vi "Handle Last Ack Core.vi"(4 "error in (no error)":errorcluster, 6 "Last Ack":refnum<class "Last Ack.lvclass">, 7 "WebSocket Service Actor in":refnum<class "WebSocket Service.lvclass">) -> (0 "error out":errorcluster, 3 "WebSocket Service Actor out":refnum<class "WebSocket Service.lvclass">)   [LabVIEW 2021, in "WebSocket Actors.lvlib" / "WebSocket Service.lvclass"]
doc: "(<B>Filename</B>: Actor Framework.lvlib:Actor.lvclass:Handle Last Ack Core.vi)\n\nDefines how the caller actor responds to the Last Ack message from a nested actor. The Last Ack message is the final message a nested actor sends to its caller before it shuts down. The message contains information about the final state of the nested actor.\n\nBy default, this method does nothing except return any error the nested actor sent. A descendant class may override this method to define behavior."
uses:
  WebSocket Service.lvclass
  <vilib>/ActorFramework/LastAck/Last Ack.lvclass
  WebSocket Connection/WebSocket Connection.lvclass
  <vilib>/ActorFramework/LastAck/Last Ack.lvclass/Last Ack.ctl
  WebSocket Service.lvclass/WebSocket Service.ctl
  WebSocket Connection/WebSocket Connection.lvclass/WebSocket Connection.ctl
  <vilib>/ActorFramework/Report Error Msg/Report Error Msg.lvclass/Report Error Msg.ctl
  <vilib>/ActorFramework/Message Enqueuer/Message Enqueuer.lvclass/Message Enqueuer.ctl
  WebSocket Connection/properties/Read Peer ID.vi
  <vilib>/ActorFramework/Message Enqueuer/Enqueue.vi
  <vilib>/ActorFramework/Report Error Msg/Report Error Msg.lvclass
  C:/Program Files/National Instruments/LabVIEW 2021/vi.lib/ActorFramework/Message/Message.lvclass
  <vilib>/Utility/LVClass/Get LV Class Name.vi
  <resource>/AFDebug/Generate Trace for Message.vi
  <vilib>/ActorFramework/Message Priority Queue/Priority Enqueue.vi
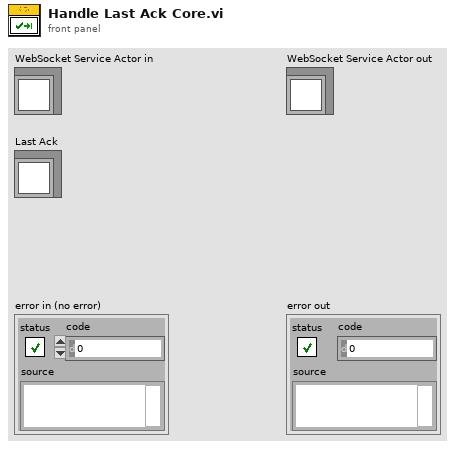
[diagram p1: front panel]
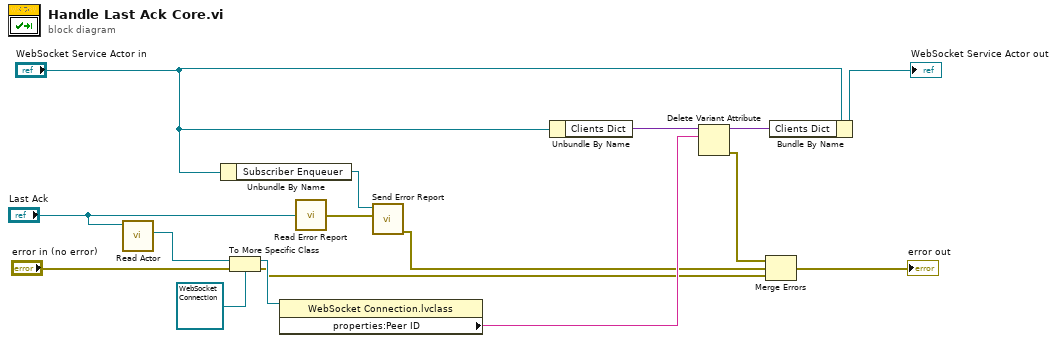
[diagram p0: block diagram]
diagram:
  n1 = call <vilib>:"Read Actor.vi"("Last Ack"="Last Ack") -> ("Actor"=w16:refnum<class "Actor.lvclass">)  [unwired: 10 in]
  n2 = Unbundle By Name("WebSocket Service Actor in") -> ("Subscriber Enqueuer"=w4:refnum<class "Message Enqueuer.lvclass">)
  n3 = To More Specific Class(target class=refnum<class "WebSocket Connection.lvclass"> refnum ("WebSocket Actors.lvlib:WebSocket Connection.lvclass"), reference=w16, error in="error in (no error)") -> (specific class reference=w15:refnum<class "WebSocket Connection.lvclass">, error out=w8:errorcluster)
  n4 = property class="WebSocket Connection.lvclass"(reference=w15) -> ("properties:Peer ID"=w9:string)  [unwired: 1 in, 2 out]
  n5 = call <vilib>:"Read Error Report.vi"("Last Ack"="Last Ack") -> ("error report"=w5:errorcluster)
  n6 = call <vilib>:"Send Error Report.vi"("Error From Sender"=w5, "Message Enqueuer"=w4) -> ("error out"=w3:errorcluster)  [unwired: 9 in]
  n7 = Unbundle By Name("WebSocket Service Actor in") -> ("Clients Dict"=w11:variant)
  n8 = Delete Variant Attribute(6:w9, 7:w11) -> (0:w2:errorcluster, 3:w10:variant)  [unwired: 1 in, 1 out]
  n9 = Merge Errors(w2, w3, w8) -> (→"error out":errorcluster)
  n10 = Bundle By Name(cluster="WebSocket Service Actor in", "Clients Dict"=w10) -> (→"WebSocket Service Actor out":refnum<class "WebSocket Service.lvclass">)
